vi "Converter Queue Driver.vi"(0 "Queue Name":string, 5 "State":T2, 7 "States[]":T2[](array[typedef]), 11 "error in (no error)":errorcluster, 13 "Operation":T1) -> (4 "Dequeued Element":T2, 15 "error out":errorcluster)   [LabVIEW 2021]
doc: "This VI acts as a queue driver for Analog To Digital Convertor VI which handles queue operations."
uses:
  Controls/State Cluster.ctl
  Controls/Queue Operation.ctl
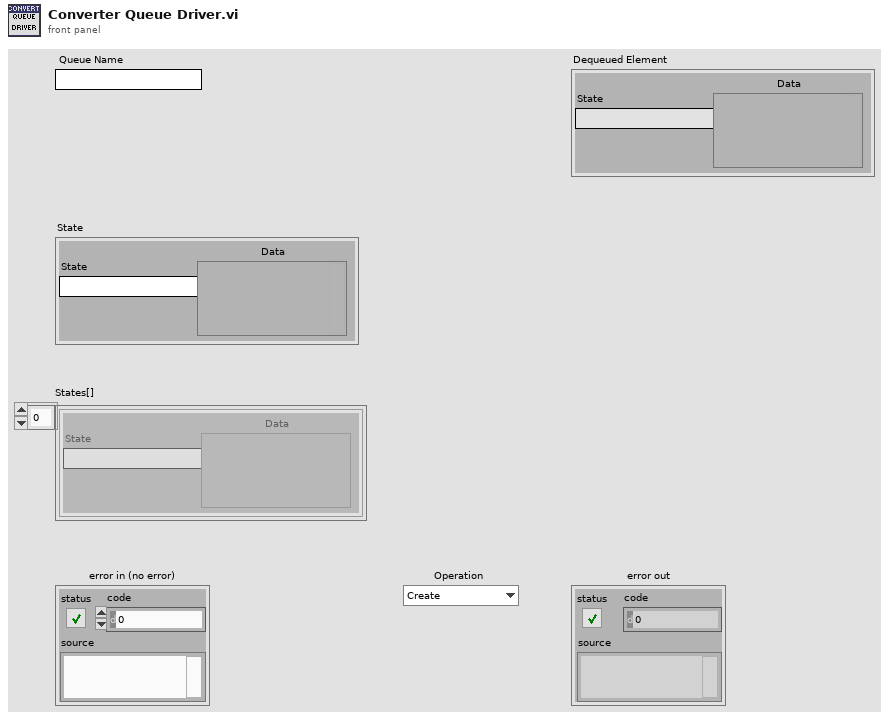
[diagram p1: front panel]
types:
  T1 = typedef "Queue Operation.ctl" = enum16{"Create", "Enqueue", "Enqueue N", "Enstack", "Dequeue", "Flush", "Release"}
  T2 = typedef "State Cluster.ctl" = cluster{"State":string, "Data":variant}
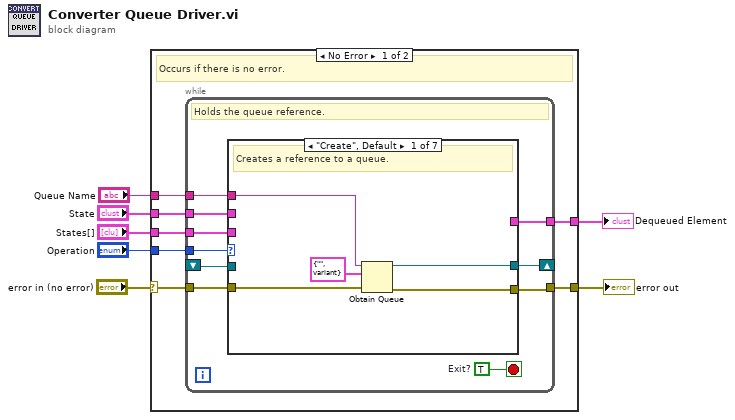
[diagram p0: block diagram]
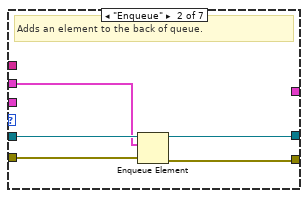
[diagram p2: hidden frame]
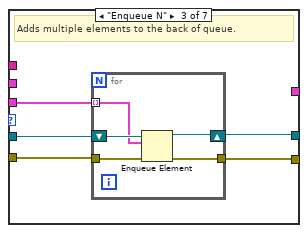
[diagram p3: hidden frame]
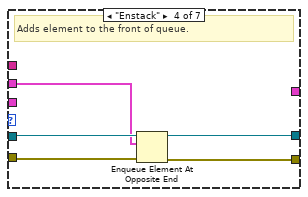
[diagram p4: hidden frame]
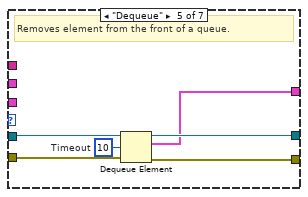
[diagram p5: hidden frame]
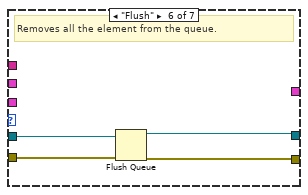
[diagram p6: hidden frame]
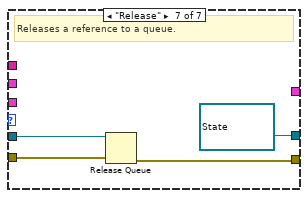
[diagram p7: hidden frame]
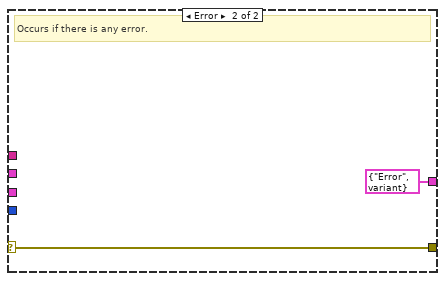
[diagram p8: hidden frame]
diagram:
  n1 = case shown="No Error" "error in (no error)" {
    selector: "error in (no error)" -> [w14 w65]
    tunnel: [w13 w65] -> w6
    tunnel: "Operation" -> [w12 _]
    tunnel: "Queue Name" -> [w11 _]
    tunnel: "State" -> [w10 _]
    tunnel: "States[]" -> [w9 _]
    tunnel: [w8 T2 {"State"="Error", "Data"=variant} ("State")] -> w1
    frame No Error {
      # "Occurs if there is no error."
      n2 = while {
        tunnel: w12 -> [w23]
        tunnel: w11 -> [w21]
        shift-right: [w20] -> _
        shift-left: _ -> [w19]
        tunnel: w10 -> [w18]
        tunnel: w9 -> [w17]
        tunnel: [w16] -> w8
        tunnel: w14 -> [w24]
        tunnel: [w22] -> w13
        stop <- w15 stop-if-true
        w15 = TRUE  # Exit?
        # "Holds the queue reference."
        n3 = case shown="\"Create\", Default" w23 {
          tunnel: w24 -> [w29 w34 w39 w49 w55 w59 w63]
          tunnel: [w28 w33 w38 w48 w54 w58 w62] -> w22
          tunnel: w21 -> [w27 _ _ _ _ _ _]
          tunnel: [w25 w30 w36 w45 w52 w56 refnum<queue> refnum ("queue out")] -> w20
          tunnel: w19 -> [_ w32 w37 w47 w53 w57 w61]
          tunnel: w18 -> [_ w31 _ w46 _ _ _]
          tunnel: w17 -> [_ _ w35 _ _ _ _]
          tunnel: [_ _ _ _ w51 _ _] -> w16
          frame "Create", Default {
            # "Creates a reference to a queue."
            n4 = Obtain Queue(name (unnamed)=w27, element data type=T2 {"State"="", "Data"=variant} ("State"), error in (no error)=w29) -> (queue out=w25:refnum<queue>, error out=w28:errorcluster)  [unwired: 2 in, 1 out]
          }
          frame "Enqueue" {
            # "Adds an element to the back of queue."
            n5 = Enqueue Element(queue=w32, element=w31, error in (no error)=w34) -> (queue out=w30:refnum<queue>, error out=w33:errorcluster)  [unwired: 1 in, 1 out]
          }
          frame "Enqueue N" {
            # "Adds multiple elements to the back of queue."
            n6 = for {
              shift-right: [w41] -> w36
              shift-left: w37 -> [w42]
              tunnel: w35 -> [w40] mode=indexing
              tunnel: w39 -> [w44]
              tunnel: [w43] -> w38
              n7 = Enqueue Element(queue=w42, element=w40, error in (no error)=w44) -> (queue out=w41:refnum<queue>, error out=w43:errorcluster)  [unwired: 1 in, 1 out]
            }
          }
          frame "Enstack" {
            # "Adds element to the front of queue."
            n8 = Enqueue Element At Opposite End(queue=w47, element=w46, error in (no error)=w49) -> (queue out=w45:refnum<queue>, error out=w48:errorcluster)  [unwired: 1 in, 1 out]
          }
          frame "Dequeue" {
            w50 = 10  # Timeout
            # "Removes element from the front of a queue."
            n9 = Dequeue Element(queue=w53, timeout in ms (-1)=w50, error in (no error)=w55) -> (queue out=w52:refnum<queue>, element=w51:T2, error out=w54:errorcluster)  [unwired: 1 out]
          }
          frame "Flush" {
            # "Removes all the element from the queue."
            n10 = Flush Queue(queue=w57, error in (no error)=w59) -> (queue out=w56:refnum<queue>, error out=w58:errorcluster)  [unwired: 1 out]
          }
          frame "Release" {
            # "Releases a reference to a queue."
            n11 = Release Queue(queue=w61, error in (no error)=w63) -> (error out=w62:errorcluster)  [unwired: 1 in, 2 out]
          }
        }
      }
    }
    frame Error {
      # "Occurs if there is any error."
    }
  }
  "Dequeued Element" <- w1
  "error out" <- w6
